vi "GetOutputVandA.vi"(9 "回来电流":string, 10 "电压系数输入":string, 11 "回来电压":string) -> (0 "电压系数输出":dbl, 1 "实际输出电压":string, 2 "字符串":string, 3 "电压系数输出":string, 4 "回来电压":dbl, 5 "实际输出电压":dbl)   [LabVIEW 2014, in "cyy.lvlib"]
uses:
  cyy.lvlib
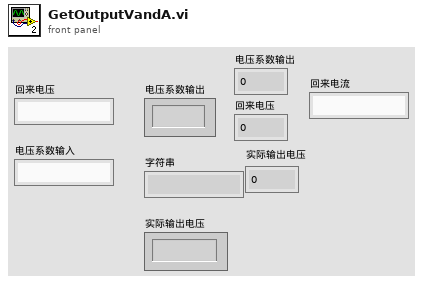
[diagram p1: front panel]
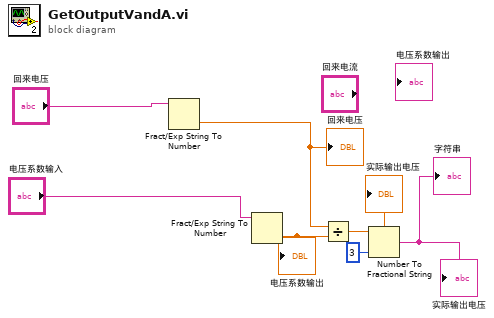
[diagram p0: block diagram]
diagram:
  n1 = Fract/Exp String To Number(string="回来电压") -> (number=w6:dbl)  [unwired: 3 in, 1 out]
  "回来电压" <- w6
  n2 = Fract/Exp String To Number(string="电压系数输入") -> (number=w1:dbl)  [unwired: 3 in, 1 out]
  "电压系数输出" <- w1
  n3 = Divide(x=w6, y=w1) -> (x/y=w7:dbl)
  "实际输出电压" <- w7
  n4 = Number To Fractional String(number=w7, precision (6)=i16 3 ("精度(6)")) -> (F-format string=→"实际输出电压" →"字符串":string)  [unwired: 2 in]
